vi "Averaging (hw2).vi"() -> ()   [LabVIEW 2017]
panel:
  in  "Knob 4":dbl(knob) scale=0.0..10.0
  in  "Knob 3":dbl(knob) scale=0.0..10.0
  in  "Knob 2":dbl(knob) scale=0.0..10.0
  in  "Knob":dbl(knob) scale=0.0..10.0
  out "Average":dbl
  # "Given 4 inputs (4 dials) you will get the average"
  # "Patrik Sokolowski"
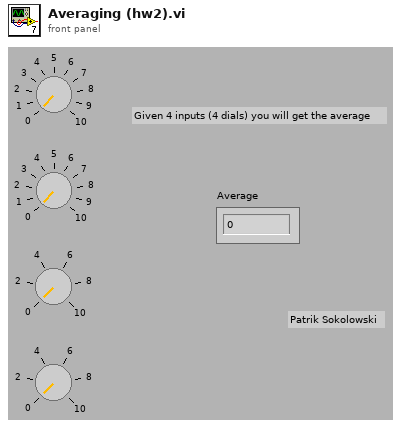
[diagram p1: front panel]
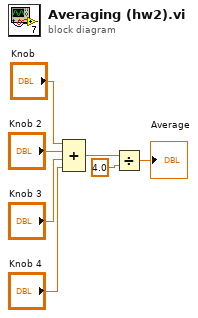
[diagram p0: block diagram]
diagram:
  n1 = Compound Arithmetic op=ADD("Knob", "Knob 2", "Knob 3", "Knob 4") -> (w3:dbl)
  n2 = Divide(x=w3, y=4.0) -> (x/y=→"Average":dbl)
